vi "Prepare.vi"(7 "Endpoint":refnum<class "Endpoint.lvclass">, 8 "error in (no error)":errorcluster, 11 "Stream in":refnum<class "Stream.lvclass">) -> (0 "error out":errorcluster, 3 "Stream out":refnum<class "Stream.lvclass">)   [LabVIEW 2020, in "Stream.lvlib" / "Stream.lvclass"]
uses:
  Stream.lvclass
  Endpoint/Endpoint.lvclass
  Stream.lvclass/Stream.ctl
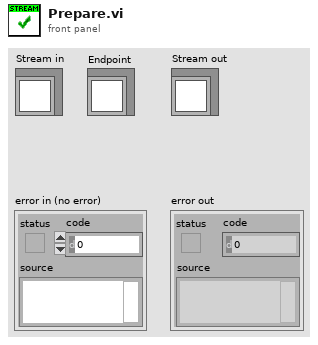
[diagram p1: front panel]
types:
  T1 = typedef "Stream.lvlib/Endpoint.lvclass/State Callback.ctl" = cluster{"Owner":refnum<class>, "VI":refnum<vi>}
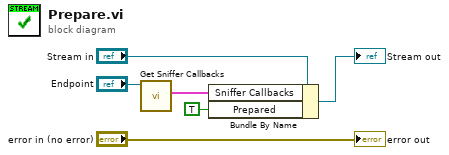
[diagram p0: block diagram]
diagram:
  n1 = call "Get Sniffer Callbacks.vi"("Endpoint in"="Endpoint") -> ("Sniffer Callbacks"=w2:T1[])  [unwired: 8 in, 2 out]
  n2 = Bundle By Name(cluster="Stream in", "Sniffer Callbacks"=w2, "Prepared"=TRUE) -> (→"Stream out":refnum<class "Stream.lvclass">)
  "error out" <- "error in (no error)"
